vi "Create Log Seg.vi"(6 "Number of Points":i32=100, 7 "Y 2":dbl(slide) scale=0.0..10.0, 8 "X 2":dbl(slide) scale=0.1..10.0, 9 "Y 1":dbl(slide) scale=0.0..10.0, 10 "X 1":dbl(slide) scale=0.1..10.0) -> (3 "Line Segment":cluster{dbl[], dbl[]}(graph))   [LabVIEW 2013]
uses:
  <vilib>/Analysis/NI_AALPro.lvlib
panel:
  in  "Sharpness":dbl(knob)=2.718281828459045 scale=0.5..1000.0
  out "error out":errorcluster
  out "Plot With Point Markers":cluster{dbl[], dbl[]}[](graph)
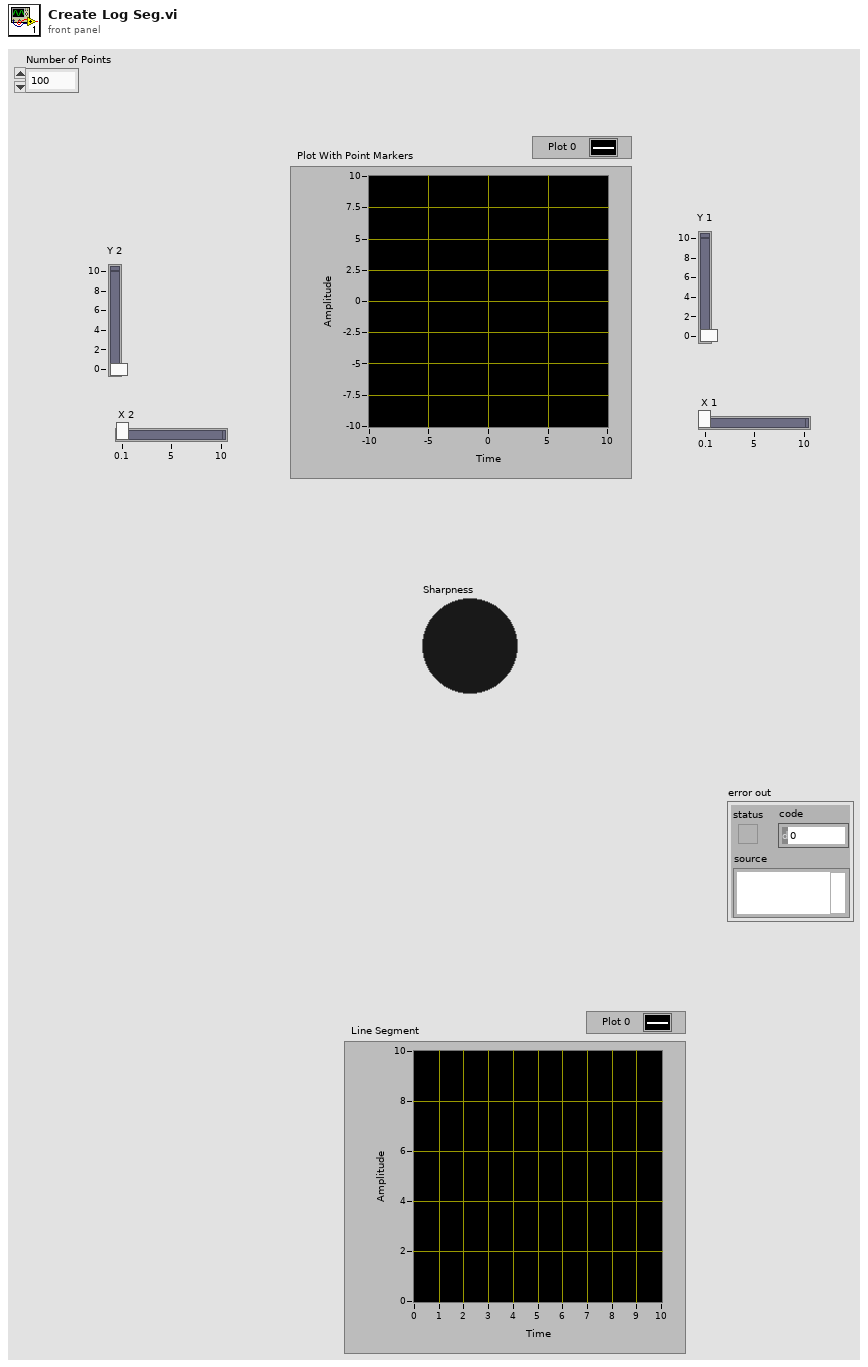
[diagram p1: front panel]
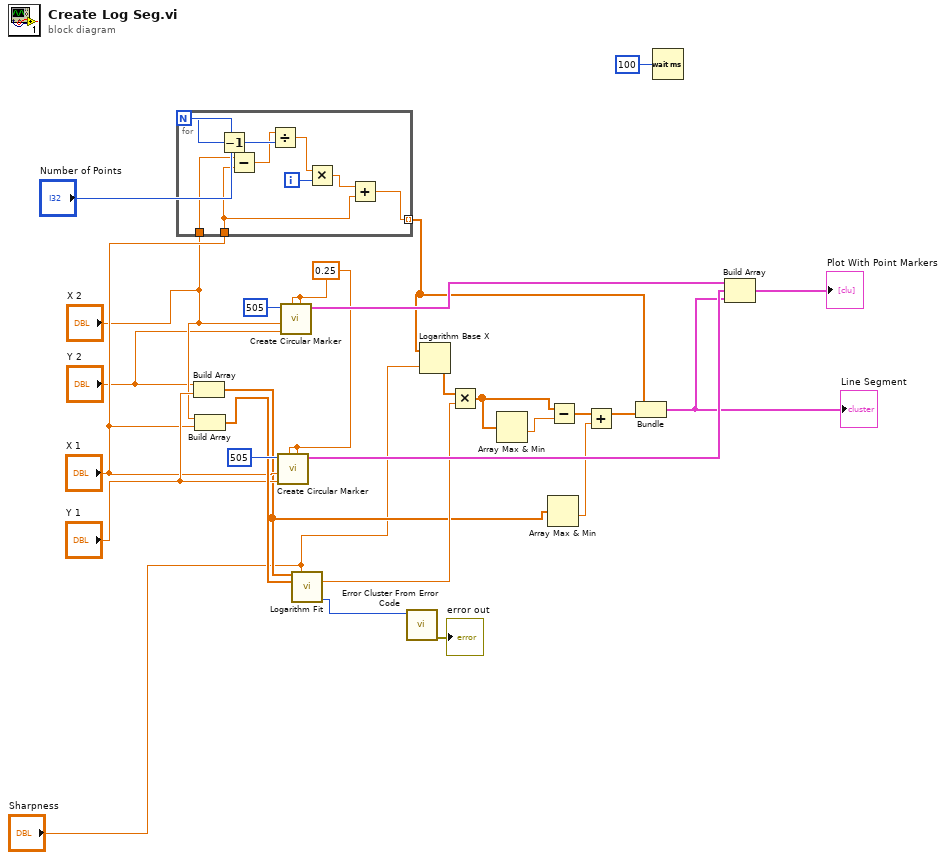
[diagram p0: block diagram]
diagram:
  w18 = 0.25 ("X Radius")
  n1 = for {
    N: "Number of Points" -> [w35]
    tunnel: [w30] -> w13 mode=indexing
    tunnel: "X 2" -> [w31]
    tunnel: "X 1" -> [w29]
    i -> [w33]
    n2 = Decrement(x=w35) -> (x-1=w28:i32)
    n3 = Subtract(x=w31, y=w29) -> (x-y=w27:dbl)
    n4 = Divide(x=w27, y=w28) -> (x/y=w34:dbl)
    n5 = Multiply(x=w34, y=w33) -> (x*y=w32:dbl)
    n6 = Add(x=w32, y=w29) -> (x+y=w30:dbl)
  }
  n7 = Build Array("Y 2", "Y 1") -> (w4:dbl[])
  n8 = Build Array("X 2", "X 1") -> (w20:dbl[])
  n9 = call "Create Circular Marker.vi"("Y Radius"=w18, "X Radius"=w18, "Y Center"="Y 1", "X Center"="X 1", "Number of Points"=505) -> ("XY Graph"=w25:cluster{dbl[], dbl[]})  [unwired: 6 in]
  n10 = call "Create Circular Marker.vi"("Y Radius"=w18, "X Radius"=w18, "Y Center"="Y 2", "X Center"="X 2", "Number of Points"=505) -> ("XY Graph"=w23:cluster{dbl[], dbl[]})  [unwired: 6 in]
  n11 = call <vilib>:"Logarithm Fit.vi"("Y"=w4, "base"="Sharpness", "X"=w20) -> ("amplitude"=w10:dbl, "error"=w17:i32)  [unwired: 8 in, 3 out]
  n12 = call <vilib>:"Error Cluster From Error Code.vi"("error code (0)"=w17) -> ("error out"=→"error out":errorcluster)  [unwired: 8 in]
  n13 = Logarithm Base X(1:"Sharpness", 2:w13) -> (0:w19:dbl[])
  n14 = Multiply(x=w19, y=w10) -> (x*y=w8:dbl[])
  n15 = Array Max & Min(array=w8) -> (min value=w9:dbl)  [unwired: 3 out]
  n16 = Array Max & Min(array=w4) -> (min value=w2:dbl)  [unwired: 3 out]
  n17 = Subtract(x=w8, y=w9) -> (x-y=w7:dbl[])
  n18 = Add(x=w7, y=w2) -> (x+y=w5:dbl[])
  n19 = Bundle(w13, w5) -> (w6:cluster{dbl[], dbl[]})  [unwired: 1 in]
  "Line Segment" <- w6
  n20 = Wait (ms)(milliseconds to wait=u32 100) -> ()  [unwired: 1 out]
  n21 = Build Array(w23, w25, w6) -> (→"Plot With Point Markers":cluster{dbl[], dbl[]}[])
